vi "GOLPI full test.vi"() -> ()   [LabVIEW 2020, in "GOLPI library.lvlib"]
doc: "Makes test of all routines in GOLPI library. Good for testing changes in GOLPI library or testing compatibility with new versions of GNU Octave."
uses:
  GOLPI library.lvlib
  Custom Error Codes Enum Type Def.vi
  Set Double.vi
  Get Double.vi
  Set Double Complex.vi
  Get Double Complex.vi
  Set 2D Array Double.vi
  Get 2D Array Double.vi
  Set 2D Array Double Complex.vi
  Get 2D Array Double Complex.vi
  Set String.vi
  Get String.vi
  Set 1D Array String.vi
  Get 1D Array String.vi
panel:
  in  "Matlab\nmode":bool
  out "file":dbl
  out "console":dbl
  in  "wait for exit\n(press this again to exit)":bool
  out "current bitstream setting":bool
  in  "hide window":bool
  out "now running test no:":i32
  out "all tests result":bool
  out "test results":T1(array[cluster])
  in  "do tests with large\nrandom datasets?":bool
  out "GNU Octave version":string
  out "exit code":i32
  out "error out":errorcluster
  in  "Octave binary directory":path=path "C:/Octave/Octave-4.0.0/bin"
  in  "Working directory":path=path "C:/"
  # "Runs various tests and checks all parts of GOLPI library.\nSelecting 'do tests with large random datasets' cause\nrunning of time consuming tests.\nIf all tests are OK, GOLPI is fully working with selected\nGNU Octave binary.\nIF WORKING DIRECTORY IS NOT WRITEABLE (C:\\ in Win7+), tests will fail also."
  # "Time consumed reading large random matrix (s)\nusing:"
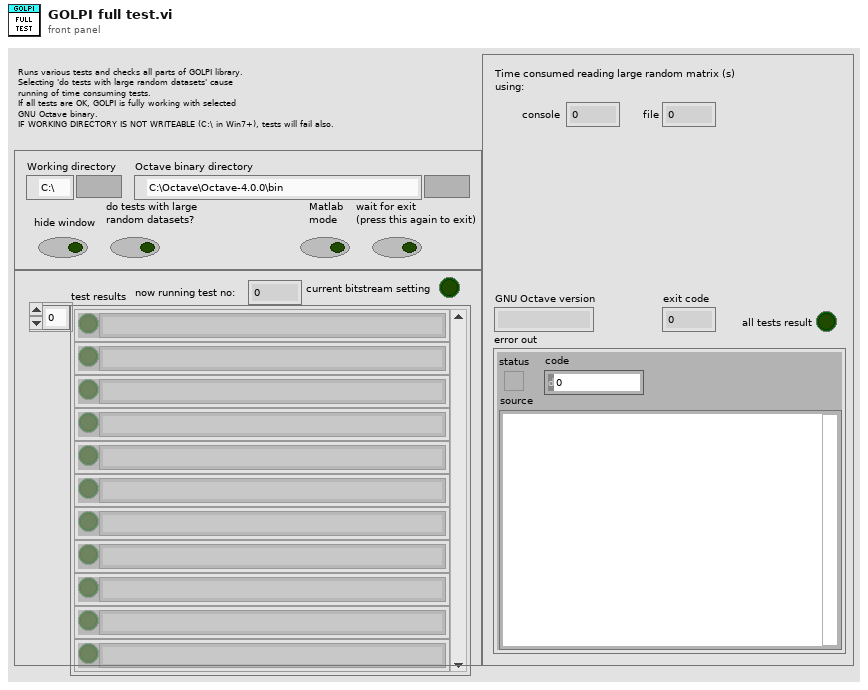
[diagram p1: front panel]
types:
  T1 = cluster{"test result":bool, "variable name":string}[]
  T2 = typedef "GOLPI library.lvlib/GOLPI reference Type Def.ctl" = cluster{"pipe handle":T3, "fast read timeout [ms]":u32, "fast read settle time [ms]":u32, "fast read to multiple [ms]":u32, "max elements per input line":u32, "slow read timeout [ms]":u32, "stdin double format specifier":string, "max elements per stdout output column":u32, "console mode bitstream":bool, "bitstream first read timeout [ms]":u32, "bitstream read timeout [ms]":u32, "struct transfer possible":bool, "matlab mode":bool}
  T3 = typedef "LV Process library.lvlib/Pipe Handle.ctl" = cluster{"lv_proc.dll file path":path, "process instance handle":u32[], "debug mode":bool, "debug data":cluster{"time":timestamp, "stdin":bool, "data":string}[]}
  T4 = typedef "GOLPI library.lvlib/Custom Error Codes Enum Type Def.vi" = enum16{"no error", "00 working directory PAR1 missing", "01 octave binary PAR1 missing", "02 octave report error PAR1", "03 empty output last cmd PAR1", "04 missing temporary file PAR1", "05 pwd PAR 1 not exist", "06 oct package not installed", "07 octave default binary missing", "10 var PAR1 not string, vect", "11 var PAR1 not num, scal, ~compl", "12 var PAR1 not num, scal, compl", "13 var PAR1 not num, vect, ~compl", "14 var PAR1 not num, vect, compl", "15 var PAR1 not num, mat, ~compl", "16 var PAR1 not num, mat, ~compl", "30 read timeout", "60 bitstream transport failed", "61 bitstream decode error PAR1", "62 bitstream cannot be set", "70 struct transfer not possible", "80 struct: cluster elem. PAR1 not implem.", "81 struct: structure field PAR1 not implem.", "82 struct: size mismatch of PAR1", "83 struct: type mismatch of PAR1", "98 internal error", "99 not finished", "90 Not supported in Matlab mode", "91 Matlab variable transfer error", "92 Matlab Script Error"}
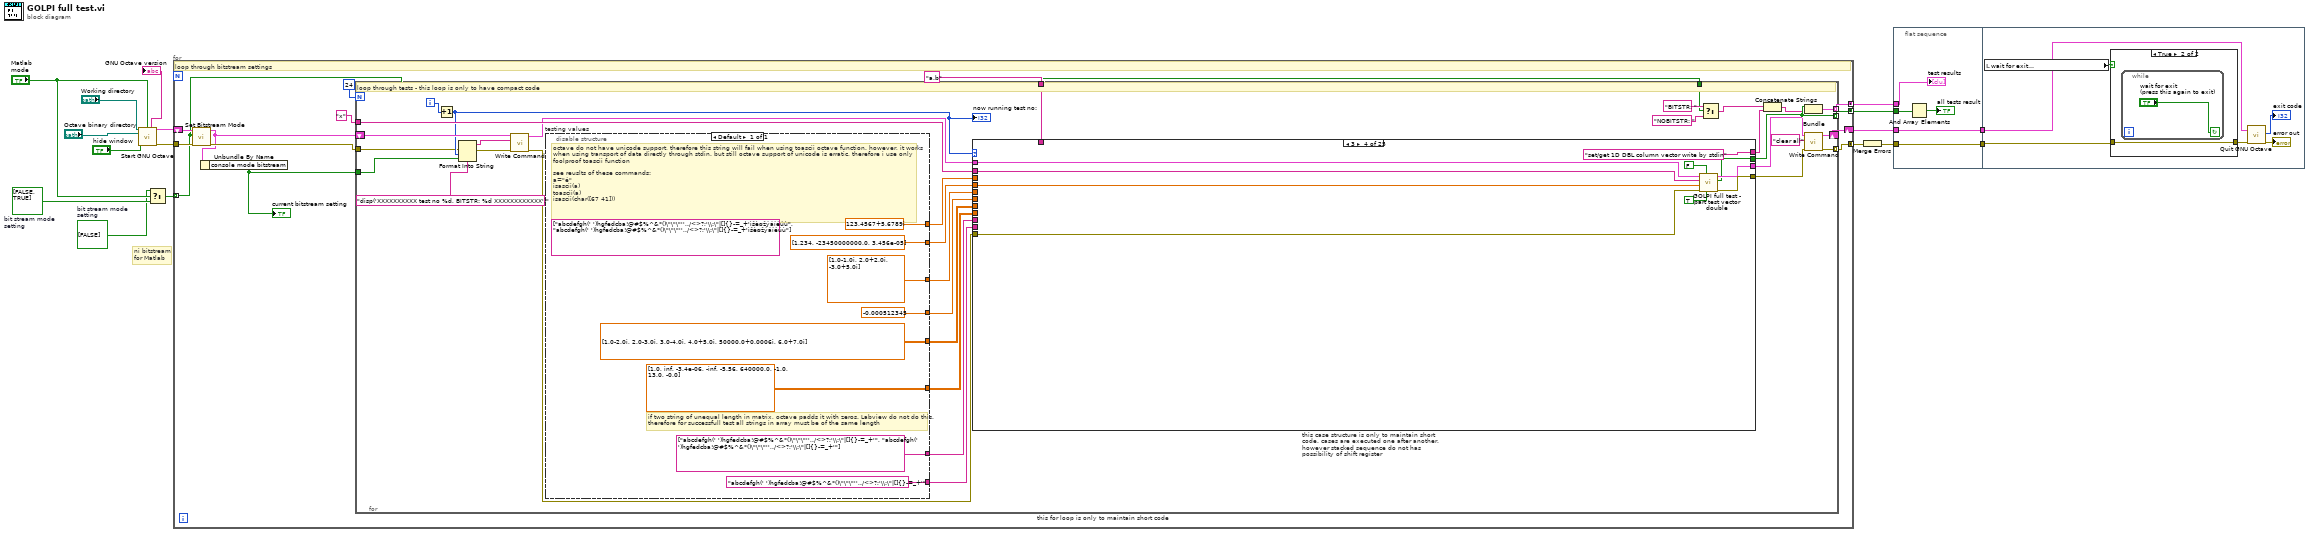
[diagram p0: block diagram]
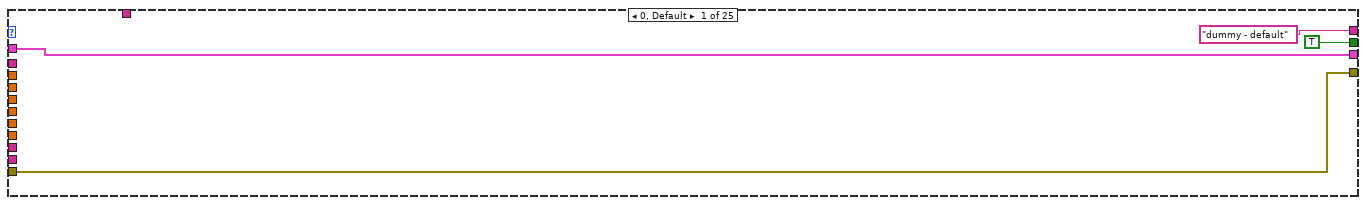
[diagram p3: hidden frame]
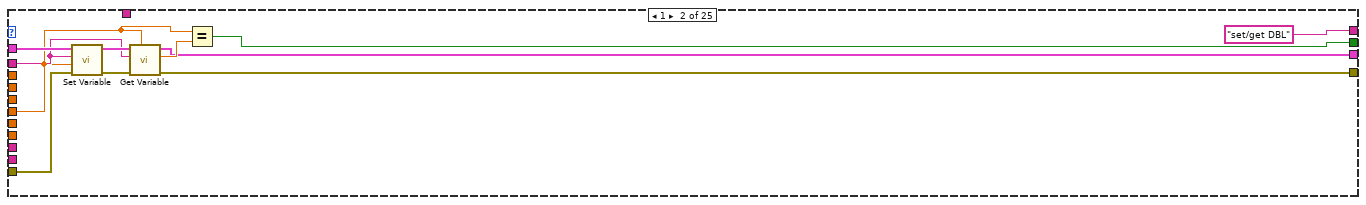
[diagram p4: hidden frame]
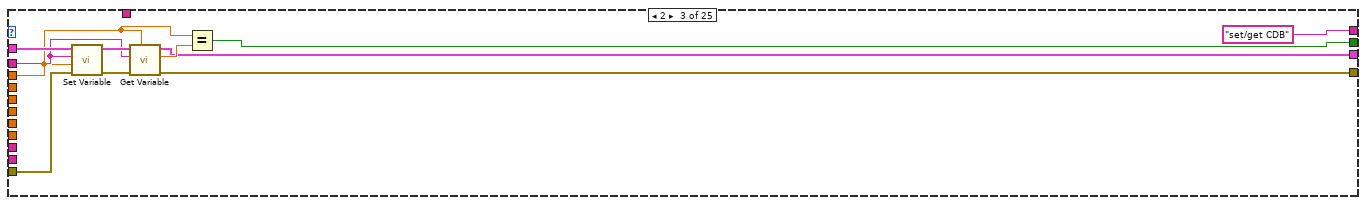
[diagram p5: hidden frame]
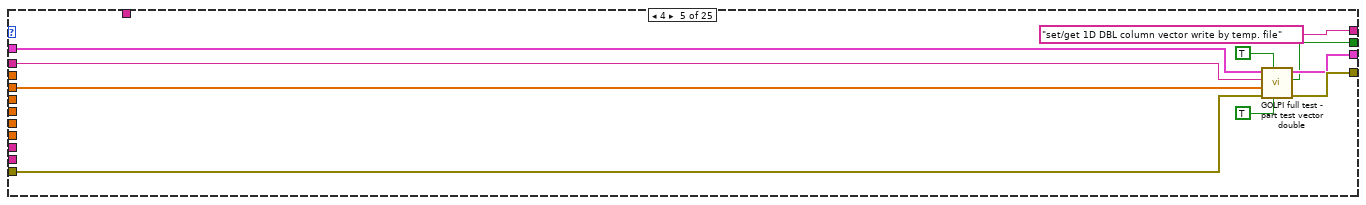
[diagram p6: hidden frame]
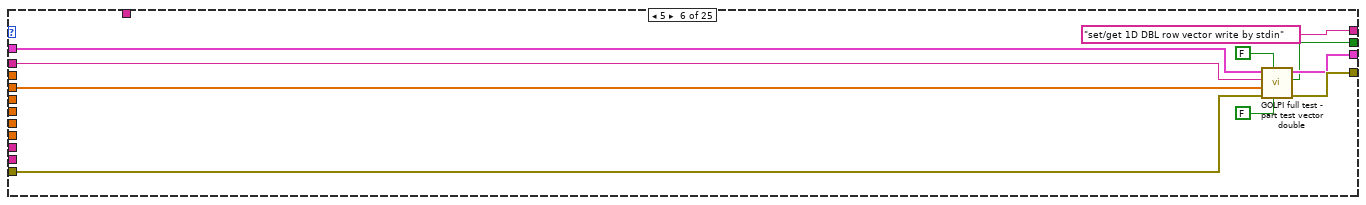
[diagram p7: hidden frame]
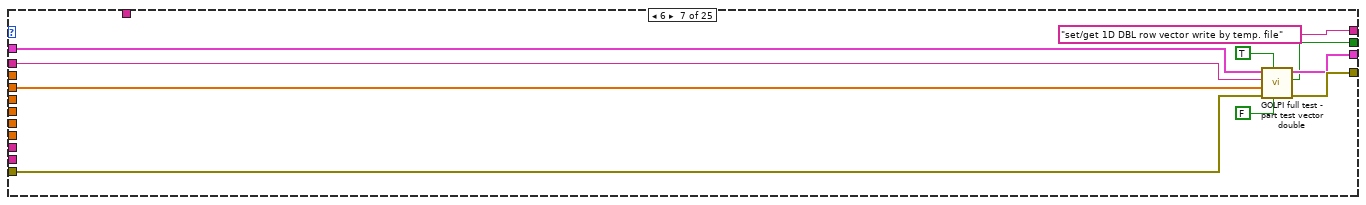
[diagram p8: hidden frame]
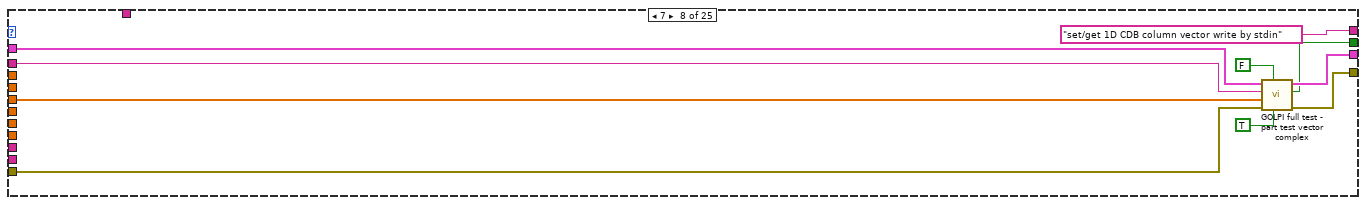
[diagram p9: hidden frame]
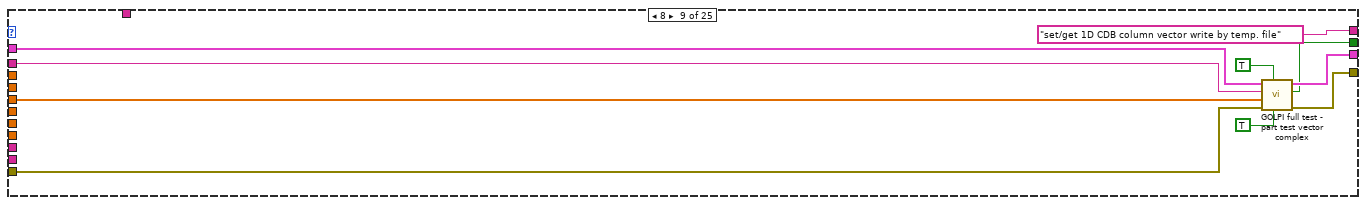
[diagram p10: hidden frame]
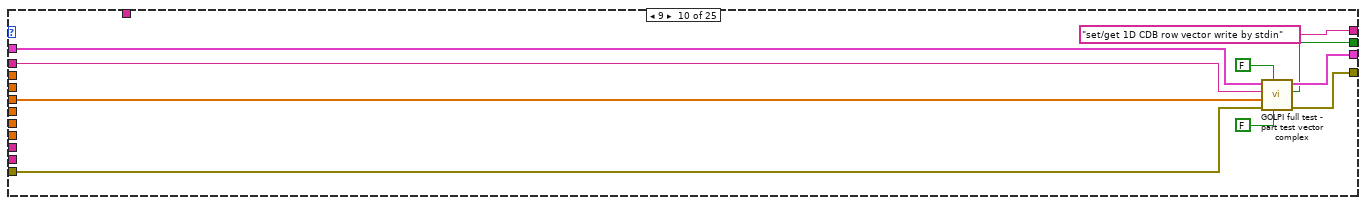
[diagram p11: hidden frame]
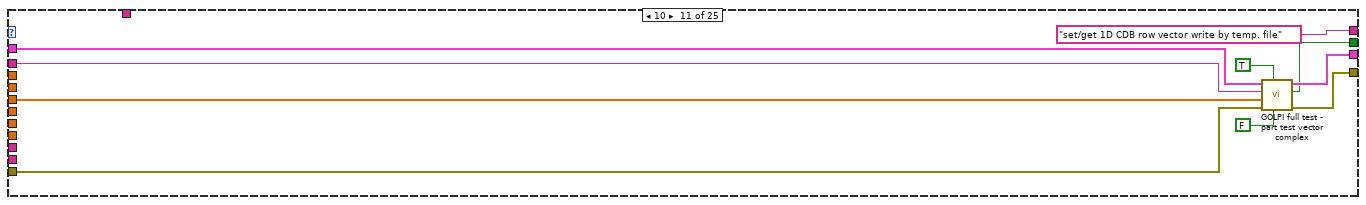
[diagram p12: hidden frame]
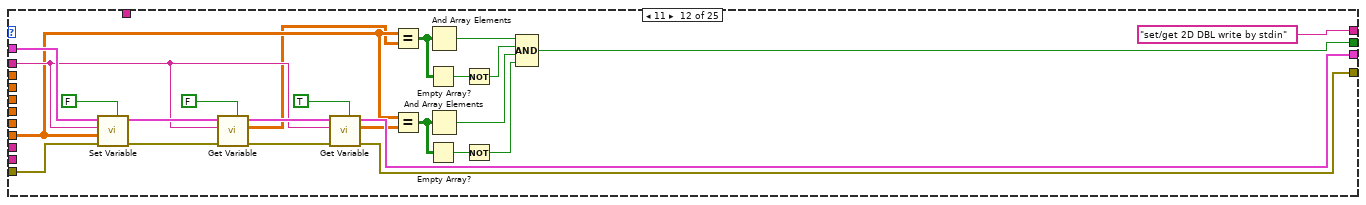
[diagram p13: hidden frame]
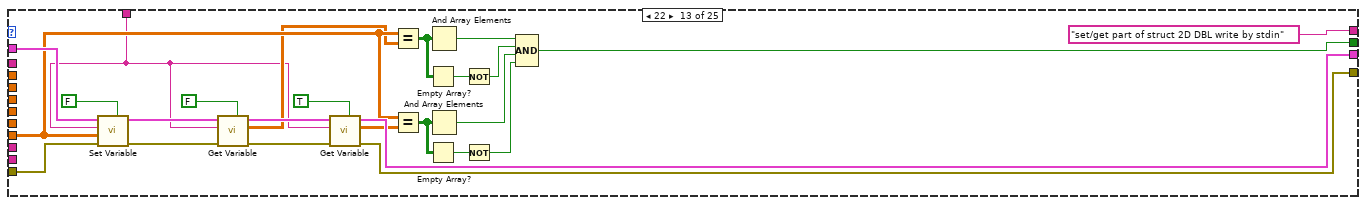
[diagram p14: hidden frame]
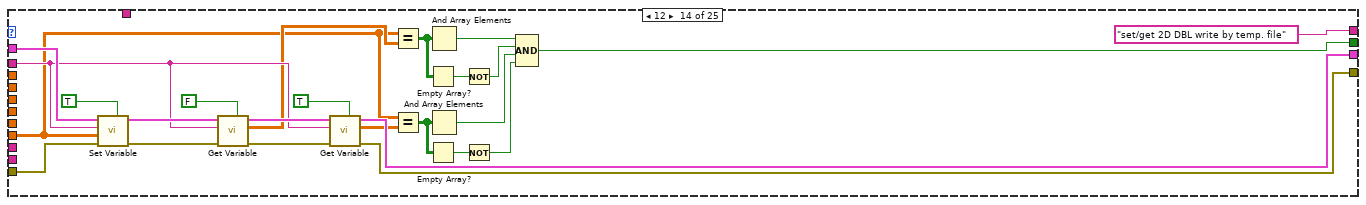
[diagram p15: hidden frame]
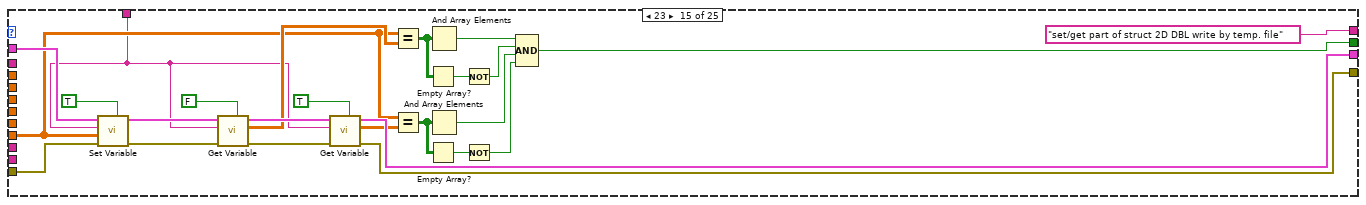
[diagram p16: hidden frame]
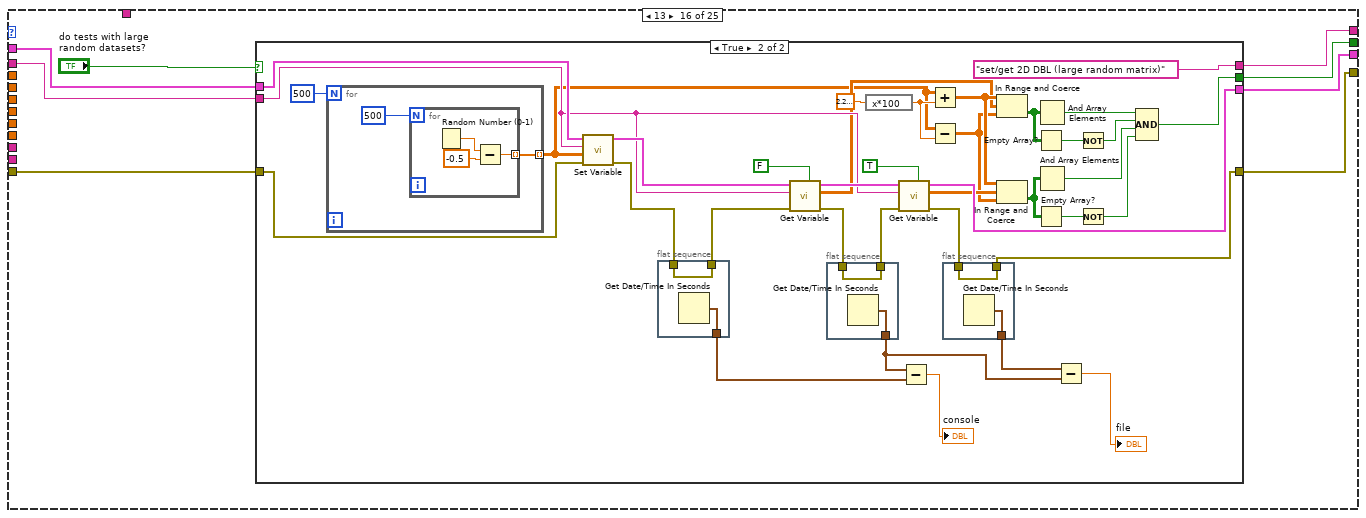
[diagram p17: hidden frame]
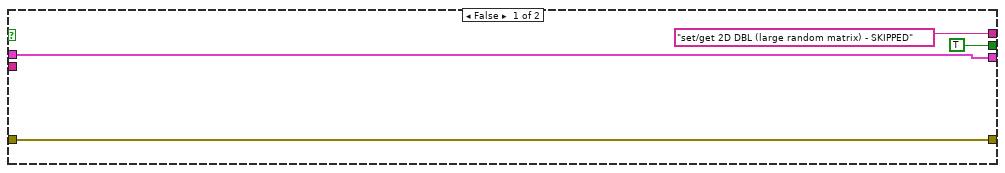
[diagram p18: hidden frame]
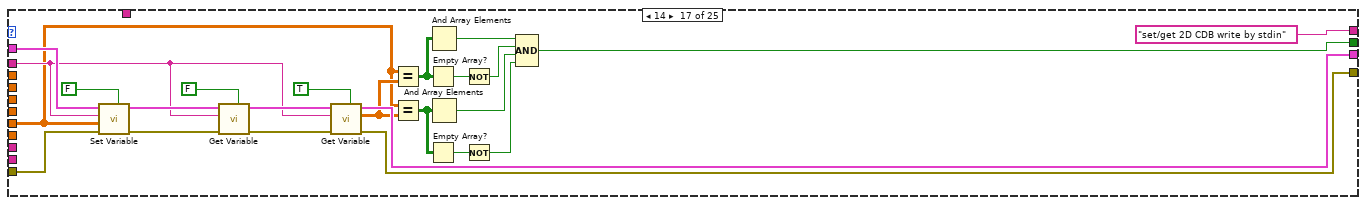
[diagram p19: hidden frame]
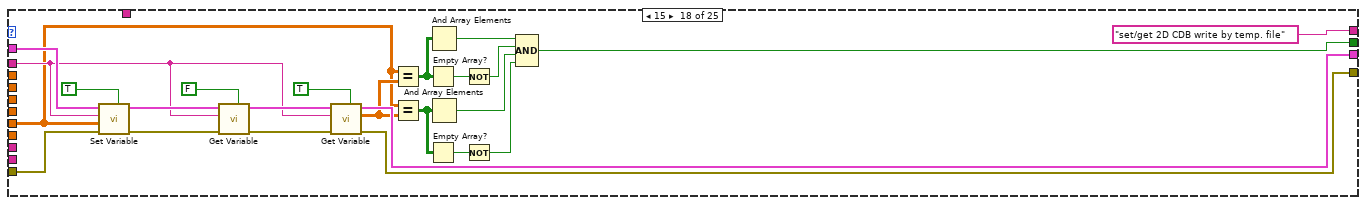
[diagram p20: hidden frame]
diagram:
  w1 = bool[] [FALSE]  # bit stream mode setting
  w2 = bool[] [FALSE, TRUE]  # bit stream mode setting
  # "ni bitstream\nfor Matlab"
  n1 = call "Start GNU Octave.vi"("working dir (user home)"="Working directory", "Matlab script mode (F)"="Matlab\nmode", "octave binary file or dir (autofind)"="Octave binary directory", "hide debug console (T)"="hide window") -> ("GNU Octave version"=→"GNU Octave version":string, "GOLPI ref. out"=w10:T2, "error out"=w15:errorcluster)  [unwired: 8 in, 1 out]
  n2 = Select(t=w1, s="Matlab\nmode", f=w2) -> (s? t:f=w4:bool[])
  n3 = for {
    tunnel: [w27] -> w14 mode=concatenating
    tunnel: [w26] -> w13 mode=concatenating
    shift-right: [w29] -> w9
    shift-left: w10 -> [w21]
    tunnel: w4 -> [w20] mode=indexing
    tunnel: w15 -> [w23]
    tunnel: [w24] -> w8 mode=concatenating
    # "loop through bitstream settings"
    n4 = call "Set Bitstream Mode.vi"("error in"=w23, "Bitstream mode (F)"=w20, "GOLPI ref. in"=w21) -> ("error out"=w22:errorcluster, "GOLPI ref. out"=w19:T2)  [unwired: 7 in]
    n5 = Unbundle By Name(w19) -> ("console mode bitstream"=w18:bool)
    "current bitstream setting" <- w18
    n6 = for "this for loop is only to maintain short code" {
      N: 24 -> [_]
      tunnel: "x" ("variable name") -> [w63]
      shift-right: [w58] -> w29
      shift-left: w19 -> [w44]
      tunnel: [w61] -> w27 mode=indexing
      tunnel: [w60] -> w26 mode=indexing
      tunnel: "a.b" ("variable name") -> [w46]
      tunnel: w20 -> [w32]
      tunnel: w18 -> [w31]
      tunnel: w22 -> [w40]
      tunnel: [w56] -> w24 mode=indexing
      i -> [w62]
      # "loop through tests - this loop is only to have compact code"
      n7 = Increment(x=w62) -> (x+1=w41:i32)
      "now running test no:" <- w41
      n8 = Format Into String(format string="disp('XXXXXXXXXX test no %d, BITSTR: %d XXXXXXXXXXXX')", error in=w40, w41, w31) -> (resulting string=w38:string, error out=w39:errorcluster)  [unwired: 1 in]
      n9 = call "Write Command.vi"("error in"=w39, "command"=w38, "GOLPI ref. in"=w44) -> ("error out"=w45:errorcluster, "GOLPI ref. out"=w43:T2)  [unwired: 7 in]
      n10 = disable-structure "testing values" shown="Default" {
        disable-tunnel: [-0.000512345 ("value")] -> w54
        disable-tunnel: [dbl[] [1.234, -23450000000.0, 3.456e-05] ("value")] -> w53
        disable-tunnel: [cdb[] [1.0-1.0i, 2.0+2.0i, -3.0+5.0i] ("value")] -> w52
        disable-tunnel: [dbl[][] [[1.0, inf, -3.4e-06], [-inf, -5.56, 640000.0], [-1.0, 13.0, -0.0]] ("value")] -> w51
        disable-tunnel: [cdb[][] [[1.0-2.0i, 2.0-3.0i, 3.0-4.0i], [4.0+5.0i, 50000.0+0.0006i, 6.0+7.0i]] ("value")] -> w50
        disable-tunnel: ["abcdefgh(' ')hgfedcba!@#$%^&*()\"\"\"'',./<>?;'\\:\"|[]{}-=_+'" ("value")] -> w49
        disable-tunnel: [string[] ["abcdefgh(' ')hgfedcba!@#$%^&*()\"\"\"'',./<>?;'\\:\"|[]{}-=_+'", "abcdefgh(' ')hgfedcba!@#$%^&*()\"\"\"'',./<>?;'\\:\"|[]{}-=_+'"]] -> w48
        disable-tunnel: [cdb 123.4567+5.6789i ("value")] -> w47
        frame Enabled {
          (unwired) string[] ["abcdefgh(' ')hgfedcba!@#$%^&*()\"\"\"'',./<>?;'\\:\"|[]{}-=_+'ìšèøžýáíéúù", "abcdefgh(' ')hgfedcba!@#$%^&*()\"\"\"'',./<>?;'\\:\"|[]{}-=_+'ìšèøžýáíéúù"]
          # "octave do not have unicode support, therefore this string will fail when using toascii octave function. however, it works\nwhen using transport of data directly through stdin. but still octave support of unicode is erratic, therefore i use only\nfoolproof toascii function\n\nsee reuslts of these commands:\na=\"é\"\nisascii(a)\ntoascii(a)\nisascii(char([67 41]))"
          # "if two string of unequal length in matrix, octave padds it with zeros. Labview do not do this.\ntherefore for successfull test all strings in array must be of the same length"
        }
      }
      n11 = case "this case structure is only to maintain short code. cases are executed one after another. however stacked sequence do not has possibility of shift register" shown="3" w41 {
        tunnel: w43 -> [w74 w83 w90 w103 w113 w125 w135 w147 w157 w164 w174 w198 w223 w248 w273 w281 w360 w384 w402 w421 w446 w471 w491 w510 w523]
        tunnel: w45 -> [w75 w82 w91 w106 w116 w127 w137 w144 w154 w167 w177 w199 w224 w249 w274 w282 w361 w385 w403 w422 w447 w472 w490 w509 w524]
        tunnel: [w75 w81 w92 w105 w115 w124 w134 w145 w155 w166 w176 w201 w226 w251 w276 w284 w359 w383 w395 w412 w434 w455 w474 w493 w516] -> w57
        tunnel: [w74 w80 w93 w104 w114 w123 w133 w146 w156 w165 w175 w200 w225 w250 w275 w283 w358 w382 w396 w410 w433 w457 w485 w505 w522] -> w59
        tunnel: w63 -> [_ w79 w89 w102 w112 w126 w136 w143 w153 w163 w173 w185 _ w235 _ w280 w340 w364 w393 w406 w432 w454 _ _ _]
        tunnel: [TRUE w78 w94 w99 w109 w122 w132 w141 w151 w160 w170 w202 w227 w252 w277 w285 w357 w381 w387 w408 w437 w462 w482 w501 w514] -> w60
        tunnel: ["dummy - default" ("variable name") "set/get DBL" ("variable name") "set/get CDB" ("variable name") "set/get 1D DBL column vector write by stdin" ("variable name") "set/get 1D DBL column vector write by temp. file" ("variable name") "set/get 1D DBL row vector write by stdin" ("variable name") "set/get 1D DBL row vector write by temp. file" ("variable name") "set/get 1D CDB column vector write by stdin" ("variable name") "set/get 1D CDB column vector write by temp. file" ("variable name") "set/get 1D CDB row vector write by stdin" ("variable name") "set/get 1D CDB row vector write by temp. file" ("variable name") "set/get 2D DBL write by stdin" ("variable name") "set/get part of struct 2D DBL write by stdin" ("variable name") "set/get 2D DBL write by temp. file" ("variable name") "set/get part of struct 2D DBL write by temp. file" ("variable name") w279 "set/get 2D CDB write by stdin" ("variable name") "set/get 2D CDB write by temp. file" ("variable name") "set/get STR write by stdin" ("variable name") "set/get STR write by temp. file" ("variable name") "set/get 1D STR write by stdin" ("variable name") "set/get 1D STR write by temp. file" ("variable name") "test read to settle" ("variable name") "test read to keyword" ("variable name") "read struct" ("variable name")] -> w34
        tunnel: w54 -> [_ w76 _ _ _ _ _ _ _ _ _ _ _ _ _ _ _ _ _ _ _ _ _ _ _]
        tunnel: w47 -> [_ _ w87 _ _ _ _ _ _ _ _ _ _ _ _ _ _ _ _ _ _ _ _ _ _]
        tunnel: w53 -> [_ _ _ w98 w108 w118 w128 _ _ _ _ _ _ _ _ _ _ _ _ _ _ _ _ _ _]
        tunnel: w52 -> [_ _ _ _ _ _ _ w138 w148 w158 w168 _ _ _ _ _ _ _ _ _ _ _ _ _ _]
        tunnel: w51 -> [_ _ _ _ _ _ _ _ _ _ _ w180 w206 w228 w254 _ _ _ _ _ _ _ _ _ _]
        tunnel: w50 -> [_ _ _ _ _ _ _ _ _ _ _ _ _ _ _ _ w338 w362 _ _ _ _ _ _ _]
        tunnel: w49 -> [_ _ _ _ _ _ _ _ _ _ _ _ _ _ _ _ _ _ w386 w405 _ _ _ _ _]
        tunnel: w48 -> [_ _ _ _ _ _ _ _ _ _ _ _ _ _ _ _ _ _ _ _ w424 w449 _ _ _]
        tunnel: w46 -> [_ _ _ _ _ _ _ _ _ _ _ _ w203 _ w253 _ _ _ _ _ _ _ _ _ _]
        frame 0, Default {
        }
        frame 1 {
          n12 = call-poly "Set Variable.vi"("error in"=w82, "value"=w76, "variable name"=w79, "GOLPI ref. in"=w83) -> ("error out"=w85:errorcluster, "GOLPI ref. out"=w86:T2)  [unwired: 6 in]
          n13 = call-poly "Get Variable.vi"("data type of variable"=w76, "error in"=w85, "variable name"=w79, "GOLPI ref. in"=w86) -> ("error out"=w81:errorcluster, "value"=w84:dbl, "GOLPI ref. out"=w80:T2)  [unwired: 5 in]
          n14 = Equal?(x=w76, y=w84) -> (x = y?=w78:bool)
        }
        frame 2 {
          n15 = call-poly "Set Variable.vi"("error in"=w91, "value"=w87, "variable name"=w89, "GOLPI ref. in"=w90) -> ("error out"=w96:errorcluster, "GOLPI ref. out"=w95:T2)  [unwired: 6 in]
          n16 = call-poly "Get Variable.vi"("data type of variable"=w87, "error in"=w96, "variable name"=w89, "GOLPI ref. in"=w95) -> ("error out"=w92:errorcluster, "value"=w97:cdb, "GOLPI ref. out"=w93:T2)  [unwired: 5 in]
          n17 = Equal?(x=w87, y=w97) -> (x = y?=w94:bool)
        }
        frame 3 {
          n18 = call "GOLPI full test - part test vector double.vi"("column vector?"=TRUE, "set: use temporary file?"=FALSE, "error in (no error)"=w106, "test value"=w98, "variable name in"=w102, "GOLPI ref. in"=w103) -> ("error out"=w105:errorcluster, "test result"=w99:bool, "GOLPI ref. out"=w104:T2)  [unwired: 3 in]
        }
        frame 4 {
          n19 = call "GOLPI full test - part test vector double.vi"("column vector?"=TRUE, "set: use temporary file?"=TRUE, "error in (no error)"=w116, "test value"=w108, "variable name in"=w112, "GOLPI ref. in"=w113) -> ("error out"=w115:errorcluster, "test result"=w109:bool, "GOLPI ref. out"=w114:T2)  [unwired: 3 in]
        }
        frame 5 {
          n20 = call "GOLPI full test - part test vector double.vi"("column vector?"=FALSE, "set: use temporary file?"=FALSE, "error in (no error)"=w127, "test value"=w118, "variable name in"=w126, "GOLPI ref. in"=w125) -> ("error out"=w124:errorcluster, "test result"=w122:bool, "GOLPI ref. out"=w123:T2)  [unwired: 3 in]
        }
        frame 6 {
          n21 = call "GOLPI full test - part test vector double.vi"("column vector?"=FALSE, "set: use temporary file?"=TRUE, "error in (no error)"=w137, "test value"=w128, "variable name in"=w136, "GOLPI ref. in"=w135) -> ("error out"=w134:errorcluster, "test result"=w132:bool, "GOLPI ref. out"=w133:T2)  [unwired: 3 in]
        }
        frame 7 {
          n22 = call "GOLPI full test - part test vector complex.vi"("column vector?"=TRUE, "set: use temporary file?"=FALSE, "error in (no error)"=w144, "test value"=w138, "variable name in"=w143, "GOLPI ref. in"=w147) -> ("error out"=w145:errorcluster, "test result"=w141:bool, "GOLPI ref. out"=w146:T2)  [unwired: 3 in]
        }
        frame 8 {
          n23 = call "GOLPI full test - part test vector complex.vi"("column vector?"=TRUE, "set: use temporary file?"=TRUE, "error in (no error)"=w154, "test value"=w148, "variable name in"=w153, "GOLPI ref. in"=w157) -> ("error out"=w155:errorcluster, "test result"=w151:bool, "GOLPI ref. out"=w156:T2)  [unwired: 3 in]
        }
        frame 9 {
          n24 = call "GOLPI full test - part test vector complex.vi"("column vector?"=FALSE, "set: use temporary file?"=FALSE, "error in (no error)"=w167, "test value"=w158, "variable name in"=w163, "GOLPI ref. in"=w164) -> ("error out"=w166:errorcluster, "test result"=w160:bool, "GOLPI ref. out"=w165:T2)  [unwired: 3 in]
        }
        frame 10 {
          n25 = call "GOLPI full test - part test vector complex.vi"("column vector?"=FALSE, "set: use temporary file?"=TRUE, "error in (no error)"=w177, "test value"=w168, "variable name in"=w173, "GOLPI ref. in"=w174) -> ("error out"=w176:errorcluster, "test result"=w170:bool, "GOLPI ref. out"=w175:T2)  [unwired: 3 in]
        }
        frame 11 {
          n26 = call-poly "Set Variable.vi"("use temporary file? (F)"=FALSE ("use temporary file?"), "error in"=w199, "value"=w180, "variable name"=w185, "GOLPI ref. in"=w198) -> ("error out"=w189:errorcluster, "GOLPI ref. out"=w187:T2)  [unwired: 5 in]
          n27 = call-poly "Get Variable.vi"("use temporary file? (F)"=FALSE ("use temporary file?"), "error in"=w189, "variable name"=w185, "GOLPI ref. in"=w187) -> ("error out"=w188:errorcluster, "value"=w179:dbl[][], "GOLPI ref. out"=w186:T2)  [unwired: 5 in]
          n28 = call-poly "Get Variable.vi"("use temporary file? (F)"=TRUE ("use temporary file?"), "error in"=w188, "variable name"=w185, "GOLPI ref. in"=w186) -> ("error out"=w201:errorcluster, "value"=w191:dbl[][], "GOLPI ref. out"=w200:T2)  [unwired: 5 in]
          n29 = Equal?(x=w180, y=w179) -> (x = y?=w178:bool[][])
          n30 = Equal?(x=w180, y=w191) -> (x = y?=w193:bool[][])
          n31 = Empty Array?(array=w178) -> (empty?=w183:bool)
          n32 = Empty Array?(array=w193) -> (empty?=w194:bool)
          n33 = And Array Elements(Boolean array=w178) -> (logical AND=w184:bool)
          n34 = And Array Elements(Boolean array=w193) -> (logical AND=w196:bool)
          n35 = Not(x=w183) -> (.not. x?=w182:bool)
          n36 = Not(x=w194) -> (.not. x?=w195:bool)
          n37 = Compound Arithmetic op=AND(w184, w182, w196, w195) -> (w202:bool)
        }
        frame 22 {
          n38 = call-poly "Set Variable.vi"("use temporary file? (F)"=FALSE ("use temporary file?"), "error in"=w224, "value"=w206, "variable name"=w203, "GOLPI ref. in"=w223) -> ("error out"=w214:errorcluster, "GOLPI ref. out"=w212:T2)  [unwired: 5 in]
          n39 = call-poly "Get Variable.vi"("use temporary file? (F)"=FALSE ("use temporary file?"), "error in"=w214, "variable name"=w203, "GOLPI ref. in"=w212) -> ("error out"=w213:errorcluster, "value"=w205:dbl[][], "GOLPI ref. out"=w211:T2)  [unwired: 5 in]
          n40 = call-poly "Get Variable.vi"("use temporary file? (F)"=TRUE ("use temporary file?"), "error in"=w213, "variable name"=w203, "GOLPI ref. in"=w211) -> ("error out"=w226:errorcluster, "value"=w216:dbl[][], "GOLPI ref. out"=w225:T2)  [unwired: 5 in]
          n41 = Equal?(x=w206, y=w205) -> (x = y?=w204:bool[][])
          n42 = Equal?(x=w206, y=w216) -> (x = y?=w218:bool[][])
          n43 = Empty Array?(array=w204) -> (empty?=w209:bool)
          n44 = Empty Array?(array=w218) -> (empty?=w219:bool)
          n45 = And Array Elements(Boolean array=w204) -> (logical AND=w210:bool)
          n46 = And Array Elements(Boolean array=w218) -> (logical AND=w221:bool)
          n47 = Not(x=w209) -> (.not. x?=w208:bool)
          n48 = Not(x=w219) -> (.not. x?=w220:bool)
          n49 = Compound Arithmetic op=AND(w210, w208, w221, w220) -> (w227:bool)
        }
        frame 12 {
          n50 = call-poly "Set Variable.vi"("use temporary file? (F)"=TRUE ("use temporary file?"), "error in"=w249, "value"=w228, "variable name"=w235, "GOLPI ref. in"=w248) -> ("error out"=w239:errorcluster, "GOLPI ref. out"=w237:T2)  [unwired: 5 in]
          n51 = call-poly "Get Variable.vi"("use temporary file? (F)"=FALSE ("use temporary file?"), "error in"=w239, "variable name"=w235, "GOLPI ref. in"=w237) -> ("error out"=w238:errorcluster, "value"=w233:dbl[][], "GOLPI ref. out"=w236:T2)  [unwired: 5 in]
          n52 = call-poly "Get Variable.vi"("use temporary file? (F)"=TRUE ("use temporary file?"), "error in"=w238, "variable name"=w235, "GOLPI ref. in"=w236) -> ("error out"=w251:errorcluster, "value"=w241:dbl[][], "GOLPI ref. out"=w250:T2)  [unwired: 5 in]
          n53 = Equal?(x=w228, y=w233) -> (x = y?=w234:bool[][])
          n54 = Equal?(x=w228, y=w241) -> (x = y?=w243:bool[][])
          n55 = Empty Array?(array=w234) -> (empty?=w231:bool)
          n56 = Empty Array?(array=w243) -> (empty?=w244:bool)
          n57 = And Array Elements(Boolean array=w234) -> (logical AND=w232:bool)
          n58 = And Array Elements(Boolean array=w243) -> (logical AND=w246:bool)
          n59 = Not(x=w231) -> (.not. x?=w230:bool)
          n60 = Not(x=w244) -> (.not. x?=w245:bool)
          n61 = Compound Arithmetic op=AND(w232, w230, w246, w245) -> (w252:bool)
        }
        frame 23 {
          n62 = call-poly "Set Variable.vi"("use temporary file? (F)"=TRUE ("use temporary file?"), "error in"=w274, "value"=w254, "variable name"=w253, "GOLPI ref. in"=w273) -> ("error out"=w264:errorcluster, "GOLPI ref. out"=w262:T2)  [unwired: 5 in]
          n63 = call-poly "Get Variable.vi"("use temporary file? (F)"=FALSE ("use temporary file?"), "error in"=w264, "variable name"=w253, "GOLPI ref. in"=w262) -> ("error out"=w263:errorcluster, "value"=w259:dbl[][], "GOLPI ref. out"=w261:T2)  [unwired: 5 in]
          n64 = call-poly "Get Variable.vi"("use temporary file? (F)"=TRUE ("use temporary file?"), "error in"=w263, "variable name"=w253, "GOLPI ref. in"=w261) -> ("error out"=w276:errorcluster, "value"=w266:dbl[][], "GOLPI ref. out"=w275:T2)  [unwired: 5 in]
          n65 = Equal?(x=w254, y=w259) -> (x = y?=w260:bool[][])
          n66 = Equal?(x=w254, y=w266) -> (x = y?=w268:bool[][])
          n67 = Empty Array?(array=w260) -> (empty?=w257:bool)
          n68 = Empty Array?(array=w268) -> (empty?=w269:bool)
          n69 = And Array Elements(Boolean array=w260) -> (logical AND=w258:bool)
          n70 = And Array Elements(Boolean array=w268) -> (logical AND=w271:bool)
          n71 = Not(x=w257) -> (.not. x?=w256:bool)
          n72 = Not(x=w269) -> (.not. x?=w270:bool)
          n73 = Compound Arithmetic op=AND(w258, w256, w271, w270) -> (w277:bool)
        }
        frame 13 {
          n74 = case shown="True" "do tests with large\nrandom datasets?" {
            tunnel: [TRUE w322] -> w285
            tunnel: [w289 w295] -> w284
            tunnel: [w288 w321] -> w283
            tunnel: w282 -> [w289 w320]
            tunnel: w281 -> [w288 w319]
            tunnel: w280 -> [_ w307]
            tunnel: ["set/get 2D DBL (large random matrix) - SKIPPED" ("variable name") "set/get 2D DBL (large random matrix)" ("variable name")] -> w279
            frame False {
            }
            frame True {
              n75 = for {
                N: 500 ("dimension size") -> [_]
                tunnel: [w334] -> w301 mode=indexing
                n76 = for {
                  N: 500 ("dimension size") -> [_]
                  tunnel: [w335] -> w334 mode=indexing
                  n77 = Random Number (0-1)() -> (number: 0 to 1=w337:dbl)
                  n78 = Subtract(x=w337, y=-0.5) -> (x-y=w335:dbl)
                }
              }
              n79 = call-poly "Set Variable.vi"("error in"=w320, "value"=w301, "variable name"=w307, "GOLPI ref. in"=w319) -> ("error out"=w299:errorcluster, "GOLPI ref. out"=w314:T2)  [unwired: 6 in]
              n80 = flat-sequence {
                tunnel: [w332] -> w300
                tunnel: w299 -> [w332]
                tunnel: [w331] -> w294
                frame #0 {
                  n81 = Get Date/Time In Seconds() -> (seconds since 1Jan1904=w331:timestamp)
                }
              }
              n82 = call-poly "Get Variable.vi"("use temporary file? (F)"=FALSE ("use temporary file?"), "error in"=w300, "variable name"=w307, "GOLPI ref. in"=w314) -> ("error out"=w298:errorcluster, "value"=w306:dbl[][], "GOLPI ref. out"=w313:T2)  [unwired: 5 in]
              n83 = flat-sequence {
                tunnel: [w330] -> w297
                tunnel: w298 -> [w330]
                tunnel: [w329] -> w292
                frame #0 {
                  n84 = Get Date/Time In Seconds() -> (seconds since 1Jan1904=w329:timestamp)
                }
              }
              n85 = expression code="x*100"(2.220446049250313e-16) -> (w304:dbl)
              n86 = call-poly "Get Variable.vi"("use temporary file? (F)"=TRUE ("use temporary file?"), "error in"=w297, "variable name"=w307, "GOLPI ref. in"=w313) -> ("error out"=w296:errorcluster, "value"=w316:dbl[][], "GOLPI ref. out"=w321:T2)  [unwired: 5 in]
              n87 = Subtract(x=w292, y=w294) -> (x-y=→"console":dbl)
              n88 = Add(x=w301, y=w304) -> (x+y=w311:dbl[][])
              n89 = Subtract(x=w301, y=w304) -> (x-y=w302:dbl[][])
              n90 = flat-sequence {
                tunnel: [w328] -> w295
                tunnel: w296 -> [w328]
                tunnel: [w327] -> w293
                frame #0 {
                  n91 = Get Date/Time In Seconds() -> (seconds since 1Jan1904=w327:timestamp)
                }
              }
              n92 = In Range and Coerce(upper limit=w311, x=w306, lower limit=w302) -> (In Range?=w303:bool[][])  [unwired: 1 out]
              n93 = In Range and Coerce(upper limit=w311, x=w316, lower limit=w302) -> (In Range?=w315:bool[][])  [unwired: 1 out]
              n94 = Empty Array?(array=w303) -> (empty?=w310:bool)
              n95 = Empty Array?(array=w315) -> (empty?=w324:bool)
              n96 = And Array Elements(Boolean array=w303) -> (logical AND=w309:bool)
              n97 = And Array Elements(Boolean array=w315) -> (logical AND=w326:bool)
              n98 = Subtract(x=w293, y=w292) -> (x-y=→"file":dbl)
              n99 = Not(x=w310) -> (.not. x?=w308:bool)
              n100 = Not(x=w324) -> (.not. x?=w325:bool)
              n101 = Compound Arithmetic op=AND(w309, w308, w326, w325) -> (w322:bool)
            }
          }
        }
        frame 14 {
          n102 = call-poly "Set Variable.vi"("use temporary file? (F)"=FALSE ("use temporary file?"), "error in"=w361, "value"=w338, "variable name"=w340, "GOLPI ref. in"=w360) -> ("error out"=w348:errorcluster, "GOLPI ref. out"=w349:T2)  [unwired: 5 in]
          n103 = call-poly "Get Variable.vi"("use temporary file? (F)"=FALSE ("use temporary file?"), "error in"=w348, "variable name"=w340, "GOLPI ref. in"=w349) -> ("error out"=w346:errorcluster, "GOLPI ref. out"=w347:T2)  [unwired: 5 in, 1 out]
          n104 = call-poly "Get Variable.vi"("use temporary file? (F)"=TRUE ("use temporary file?"), "error in"=w346, "variable name"=w340, "GOLPI ref. in"=w347) -> ("error out"=w359:errorcluster, "value"=w341:cdb[][], "GOLPI ref. out"=w358:T2)  [unwired: 5 in]
          n105 = Equal?(x=w338, y=w341) -> (x = y?=w344:bool[][])
          n106 = Equal?(x=w338, y=w341) -> (x = y?=w354:bool[][])
          n107 = Empty Array?(array=w344) -> (empty?=w345:bool)
          n108 = Empty Array?(array=w354) -> (empty?=w353:bool)
          n109 = And Array Elements(Boolean array=w344) -> (logical AND=w343:bool)
          n110 = And Array Elements(Boolean array=w354) -> (logical AND=w351:bool)
          n111 = Not(x=w345) -> (.not. x?=w342:bool)
          n112 = Not(x=w353) -> (.not. x?=w352:bool)
          n113 = Compound Arithmetic op=AND(w343, w342, w351, w352) -> (w357:bool)
        }
        frame 15 {
          n114 = call-poly "Set Variable.vi"("use temporary file? (F)"=TRUE ("use temporary file?"), "error in"=w385, "value"=w362, "variable name"=w364, "GOLPI ref. in"=w384) -> ("error out"=w372:errorcluster, "GOLPI ref. out"=w373:T2)  [unwired: 5 in]
          n115 = call-poly "Get Variable.vi"("use temporary file? (F)"=FALSE ("use temporary file?"), "error in"=w372, "variable name"=w364, "GOLPI ref. in"=w373) -> ("error out"=w370:errorcluster, "GOLPI ref. out"=w371:T2)  [unwired: 5 in, 1 out]
          n116 = call-poly "Get Variable.vi"("use temporary file? (F)"=TRUE ("use temporary file?"), "error in"=w370, "variable name"=w364, "GOLPI ref. in"=w371) -> ("error out"=w383:errorcluster, "value"=w365:cdb[][], "GOLPI ref. out"=w382:T2)  [unwired: 5 in]
          n117 = Equal?(x=w362, y=w365) -> (x = y?=w368:bool[][])
          n118 = Equal?(x=w362, y=w365) -> (x = y?=w378:bool[][])
          n119 = Empty Array?(array=w368) -> (empty?=w369:bool)
          n120 = Empty Array?(array=w378) -> (empty?=w377:bool)
          n121 = And Array Elements(Boolean array=w368) -> (logical AND=w367:bool)
          n122 = And Array Elements(Boolean array=w378) -> (logical AND=w375:bool)
          n123 = Not(x=w369) -> (.not. x?=w366:bool)
          n124 = Not(x=w377) -> (.not. x?=w376:bool)
          n125 = Compound Arithmetic op=AND(w367, w366, w375, w376) -> (w381:bool)
        }
        frame 16 {
          n126 = call-poly "Set Variable.vi"("use temporary file? (F)"=FALSE ("use temporary file?"), "error in"=w403, "value"=w386, "variable name"=w393, "GOLPI ref. in"=w402) -> ("error out"=w404:errorcluster, "GOLPI ref. out"=w401:T2)  [unwired: 5 in]
          n127 = call-poly "Get Variable.vi"("use temporary file? (F)"=FALSE ("use temporary file?"), "error in"=w404, "variable name"=w393, "GOLPI ref. in"=w401) -> ("error out"=w394:errorcluster, "value"=w400:string, "GOLPI ref. out"=w397:T2)  [unwired: 5 in]
          n128 = call-poly "Get Variable.vi"("use temporary file? (F)"=TRUE ("use temporary file?"), "error in"=w394, "variable name"=w393, "GOLPI ref. in"=w397) -> ("error out"=w395:errorcluster, "value"=w390:string, "GOLPI ref. out"=w396:T2)  [unwired: 5 in]
          n129 = Equal?(x=w386, y=w400) -> (x = y?=w388:bool)
          n130 = Equal?(x=w386, y=w390) -> (x = y?=w389:bool)
          n131 = And(x=w388, y=w389) -> (x .and. y?=w387:bool)
        }
        frame 17 {
          n132 = call-poly "Set Variable.vi"("use temporary file? (F)"=TRUE ("use temporary file?"), "error in"=w422, "value"=w405, "variable name"=w406, "GOLPI ref. in"=w421) -> ("error out"=w423:errorcluster, "GOLPI ref. out"=w420:T2)  [unwired: 5 in]
          n133 = call-poly "Get Variable.vi"("use temporary file? (F)"=FALSE ("use temporary file?"), "error in"=w423, "variable name"=w406, "GOLPI ref. in"=w420) -> ("error out"=w413:errorcluster, "value"=w419:string, "GOLPI ref. out"=w411:T2)  [unwired: 5 in]
          n134 = call-poly "Get Variable.vi"("use temporary file? (F)"=TRUE ("use temporary file?"), "error in"=w413, "variable name"=w406, "GOLPI ref. in"=w411) -> ("error out"=w412:errorcluster, "value"=w415:string, "GOLPI ref. out"=w410:T2)  [unwired: 5 in]
          n135 = Equal?(x=w405, y=w419) -> (x = y?=w409:bool)
          n136 = Equal?(x=w405, y=w415) -> (x = y?=w414:bool)
          n137 = And(x=w409, y=w414) -> (x .and. y?=w408:bool)
        }
        frame 18 {
          n138 = call-poly "Set Variable.vi"("use temporary file? (F)"=FALSE ("use temporary file? 2"), "error in"=w447, "value"=w424, "variable name"=w432, "GOLPI ref. in"=w446) -> ("error out"=w448:errorcluster, "GOLPI ref. out"=w445:T2)  [unwired: 5 in]
          n139 = call-poly "Get Variable.vi"("use temporary file? (F)"=FALSE ("use temporary file?"), "error in"=w448, "variable name"=w432, "GOLPI ref. in"=w445) -> ("error out"=w435:errorcluster, "value"=w444:string[], "GOLPI ref. out"=w436:T2)  [unwired: 5 in]
          n140 = call-poly "Get Variable.vi"("use temporary file? (F)"=TRUE ("use temporary file?"), "error in"=w435, "variable name"=w432, "GOLPI ref. in"=w436) -> ("error out"=w434:errorcluster, "value"=w427:string[], "GOLPI ref. out"=w433:T2)  [unwired: 5 in]
          n141 = Equal?(x=w424, y=w444) -> (x = y?=w438:bool[])
          n142 = Equal?(x=w424, y=w427) -> (x = y?=w431:bool[])
          n143 = And Array Elements(Boolean array=w438) -> (logical AND=w441:bool)
          n144 = Empty Array?(array=w438) -> (empty?=w439:bool)
          n145 = And Array Elements(Boolean array=w431) -> (logical AND=w428:bool)
          n146 = Empty Array?(array=w431) -> (empty?=w430:bool)
          n147 = Not(x=w439) -> (.not. x?=w440:bool)
          n148 = Not(x=w430) -> (.not. x?=w429:bool)
          n149 = Compound Arithmetic op=AND(w441, w440, w428, w429) -> (w437:bool)
        }
        frame 19 {
          n150 = call-poly "Set Variable.vi"("use temporary file? (F)"=TRUE ("use temporary file? 2"), "error in"=w472, "value"=w449, "variable name"=w454, "GOLPI ref. in"=w471) -> ("error out"=w473:errorcluster, "GOLPI ref. out"=w470:T2)  [unwired: 5 in]
          n151 = call-poly "Get Variable.vi"("use temporary file? (F)"=FALSE ("use temporary file?"), "error in"=w473, "variable name"=w454, "GOLPI ref. in"=w470) -> ("error out"=w456:errorcluster, "value"=w469:string[], "GOLPI ref. out"=w458:T2)  [unwired: 5 in]
          n152 = call-poly "Get Variable.vi"("use temporary file? (F)"=TRUE ("use temporary file?"), "error in"=w456, "variable name"=w454, "GOLPI ref. in"=w458) -> ("error out"=w455:errorcluster, "value"=w450:string[], "GOLPI ref. out"=w457:T2)  [unwired: 5 in]
          n153 = Equal?(x=w449, y=w469) -> (x = y?=w463:bool[])
          n154 = Equal?(x=w449, y=w450) -> (x = y?=w459:bool[])
          n155 = And Array Elements(Boolean array=w463) -> (logical AND=w466:bool)
          n156 = Empty Array?(array=w463) -> (empty?=w464:bool)
          n157 = And Array Elements(Boolean array=w459) -> (logical AND=w453:bool)
          n158 = Empty Array?(array=w459) -> (empty?=w460:bool)
          n159 = Not(x=w464) -> (.not. x?=w465:bool)
          n160 = Not(x=w460) -> (.not. x?=w452:bool)
          n161 = Compound Arithmetic op=AND(w466, w465, w453, w452) -> (w462:bool)
        }
        frame 20 {
          # "should generate\nnot supporte\nerror"
          n162 = call "Write Command.vi"("error in"=w490, "command"="for i=[1:10]\n   pause(1)\n   disp(i)\nend", "GOLPI ref. in"=w491) -> ("error out"=w488:errorcluster, "GOLPI ref. out"=w489:T2)  [unwired: 7 in]
          n163 = call "Read Output Till Settle.vi"("timeout [ms]"=u32 13000, "error in"=w488, "settled for [ms]"=u32 1100, "GOLPI ref. in"=w489) -> ("error out"=w475:errorcluster, "GOLPI ref. out"=w485:T2)  [unwired: 4 in, 2 out]
          n164 = Unbundle By Name(w475) -> ("code"=w479:i32)
          n165 = call "Generate Custom Error.vi"("GOLPI error"=Custom_Error_Codes_Enum_Type_Def.vi."90 Not supported in Matlab mode") -> ("error out"=w481:errorcluster)  [unwired: 10 in]
          n166 = Unbundle By Name(w481) -> ("code"=w480:i32)
          n167 = Not Equal?(x=w479, y=w480) -> (x != y?=w477:bool)
          n168 = Select(t=w475, s=w477, f=errorcluster {"status"=FALSE, "code"=0, "source"=""}) -> (s? t:f=w474:errorcluster)
          n169 = Unbundle By Name(w474) -> ("status"=w483:bool)
          n170 = Not(x=w483) -> (.not. x?=w482:bool)
        }
        frame 21 {
          # "should generate\nnot supporte\nerror"
          n171 = call "Write Command.vi"("error in"=w509, "command"="for i=[1:10]\n   pause(1)\n  end\ndisp('testkeyword')", "GOLPI ref. in"=w510) -> ("error out"=w507:errorcluster, "GOLPI ref. out"=w506:T2)  [unwired: 7 in]
          n172 = call "Read Output Till Keyword.vi"("timeout [ms]"=u32 13000, "error in"=w507, "keywords"=string[] ["error", "testkeyword"], "GOLPI ref. in"=w506) -> ("error out"=w494:errorcluster, "GOLPI ref. out"=w505:T2)  [unwired: 4 in, 2 out]
          n173 = Unbundle By Name(w494) -> ("code"=w498:i32)
          n174 = call "Generate Custom Error.vi"("GOLPI error"=Custom_Error_Codes_Enum_Type_Def.vi."90 Not supported in Matlab mode") -> ("error out"=w500:errorcluster)  [unwired: 10 in]
          n175 = Unbundle By Name(w500) -> ("code"=w499:i32)
          n176 = Not Equal?(x=w498, y=w499) -> (x != y?=w496:bool)
          n177 = Select(t=w494, s=w496, f=errorcluster {"status"=FALSE, "code"=0, "source"=""}) -> (s? t:f=w493:errorcluster)
          n178 = Unbundle By Name(w493) -> ("status"=w502:bool)
          n179 = Not(x=w502) -> (.not. x?=w501:bool)
        }
        frame 24 {
          # "should generate\nnot supporte\nerror"
          n180 = call "GOLPI full test - part structure.vi"("error in"=w524, "GOLPI ref. in"=w523) -> ("error out"=w517:errorcluster, "match"=w513:bool, "GOLPI ref. out"=w522:T2)  [unwired: 7 in]
          n181 = Unbundle By Name(w517) -> ("code"=w518:i32)
          n182 = call "Generate Custom Error.vi"("GOLPI error"=Custom_Error_Codes_Enum_Type_Def.vi."90 Not supported in Matlab mode") -> ("error out"=w520:errorcluster)  [unwired: 10 in]
          n183 = Unbundle By Name(w520) -> ("code"=w519:i32)
          n184 = Not Equal?(x=w518, y=w519) -> (x != y?=w512:bool)
          n185 = Compound Arithmetic op=OR(w513, invert w512) -> (w514:bool)
          n186 = Select(t=w517, s=w512, f=errorcluster {"status"=FALSE, "code"=0, "source"=""}) -> (s? t:f=w516:errorcluster)
        }
      }
      n187 = Select(t="BITSTR: " ("variable name"), s=w32, f="NOBITSTR: " ("variable name")) -> (s? t:f=w35:string)
      n188 = Concatenate Strings(w35, w34) -> (w33:string)
      n189 = Bundle("test result"=w60, w33) -> (w61:cluster{"test result":bool, string})  [unwired: 1 in]
      n190 = call "Write Command.vi"("error in"=w57, "command"="clear all", "GOLPI ref. in"=w59) -> ("error out"=w56:errorcluster, "GOLPI ref. out"=w58:T2)  [unwired: 7 in]
    }
  }
  n191 = Merge Errors(w8) -> (w5:errorcluster)
  n192 = flat-sequence {
    tunnel: w14 -> [w530]
    tunnel: w13 -> [w529]
    tunnel: w9 -> [w526]
    tunnel: w5 -> [w527]
    tunnel: [w527] -> w7
    tunnel: [w526] -> w6
    tunnel: w7 -> [w532]
    tunnel: w6 -> [w531]
    frame #0 {
      n193 = And Array Elements(Boolean array=w529) -> (logical AND=→"all tests result":bool)
      "test results" <- w530
    }
    frame #1 {
      n194 = local read "wait for exit\n(press this again to exit)"() -> (w535:bool)
      n195 = case shown="True" w535 {
        tunnel: [w537 w538] -> w536
        tunnel: w532 -> [w537 w538]
        frame False {
        }
        frame True {
          n196 = while {
            stop <- "wait for exit\n(press this again to exit)" continue-if-true
          }
        }
      }
      n197 = call "Quit GNU Octave.vi"("error in"=w536, "GOLPI ref. in"=w531) -> ("error out"=→"error out":errorcluster, "exit code"=→"exit code":i32)  [unwired: 8 in]
    }
  }
